vi "List Roots.vi"(8 "Error In":errorcluster, 11 "Tree Manager":T1) -> (0 "Error Out":errorcluster, 1 "Roots IDs":string[](array[string]), 2 "Roots Names":string[](array[string]), 3 "Tree Manager":T1)   [LabVIEW 2016, in "Tree Manager.lvclass"]
doc: "List the Trees that have no Parent ID specified.\n\nThe list order is random."
uses:
  Tree Manager.lvclass
  Typedefs/Session Handle.ctl
  Tree Manager.lvclass/Tree Manager.ctl
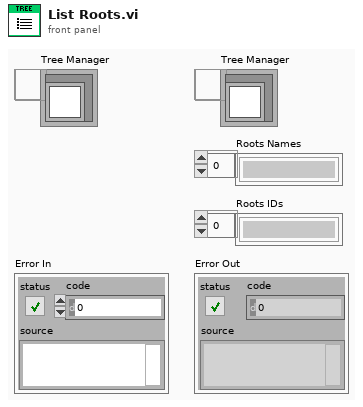
[diagram p1: front panel]
types:
  T1 = typedef "Tree Manager.lvclass/Session Handle.ctl" = refnum<data-value>
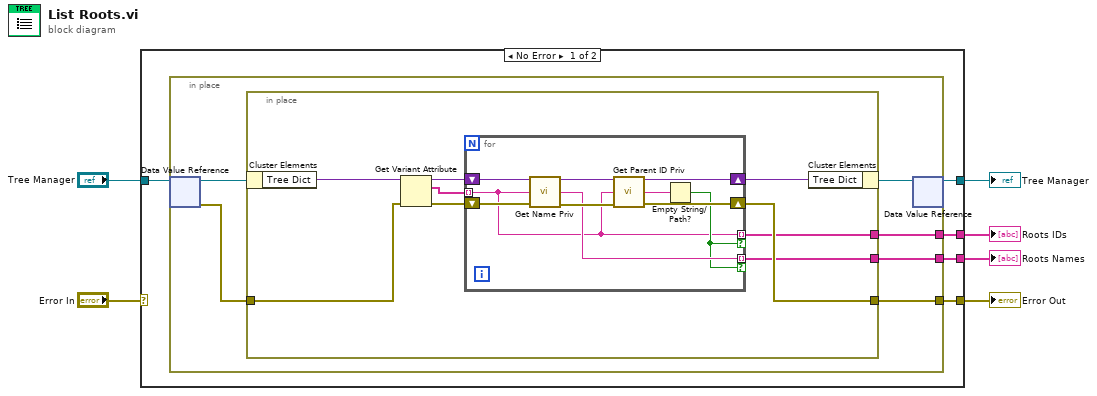
[diagram p0: block diagram]
diagram:
  n1 = case shown="No Error" "Error In" {
    selector: "Error In" -> [_ w37]
    tunnel: "Tree Manager" -> [w11 w38]
    tunnel: [w10 w38] -> w5
    tunnel: [w9 w37] -> w3
    tunnel: [w8 _] -> w2
    tunnel: [w7 _] -> w1
    frame No Error {
      n2 = in-place {
        in-place-border: [w16] -> w9
        in-place-border: [w13] -> w8
        in-place-border: [w12] -> w7
        n3 = in-place-dvr #1(w11) -> (w17:refnum<class "Tree Manager.lvclass">, w14:errorcluster)
        n4 = in-place {
          in-place-border: [w21] -> w16
          in-place-border: w14 -> [w25]
          in-place-border: [w19] -> w13
          in-place-border: [w18] -> w12
          n5 = in-place-cluster #2(w17) -> ("Tree Dict"=w26:variant)
          n6 = Get Variant Attribute(Variant=w26, error in=w25) -> (duplicate Variant=w24:variant, names=w20:string[], error out=w22:errorcluster)  [unwired: 2 in, 1 out]
          n7 = for {
            shift-right: [w36] -> w23
            shift-left: w24 -> [w33]
            shift-right: [w35] -> w21
            shift-left: w22 -> [w30]
            tunnel: w20 -> [w27] mode=indexing
            tunnel: [w27] -> w19 mode=indexing if=w28
            tunnel: [w29] -> w18 mode=indexing if=w28
            n8 = call "Get Name Priv.vi"("Tree Dictionary"=w33, "Unique ID"=w27, "error in"=w30) -> ("Tree Dictionary Out"=w32:variant, "Name"=w29:string, "error out"=w31:errorcluster)  [unwired: 10 in]
            n9 = call "Get Parent ID Priv.vi"("Tree Dictionary"=w32, "Unique ID"=w27, "error in"=w31) -> ("Tree Dictionary Out"=w36:variant, "Parent ID"=w34:string, "error out"=w35:errorcluster)  [unwired: 10 in]
            n10 = Empty String/Path?(string/path=w34) -> (empty?=w28:bool)
          }
          n11 = in-place-cluster #2("Tree Dict"=w23) -> (w15:refnum<class "Tree Manager.lvclass">)
        }
        n12 = in-place-dvr #1(w15) -> (w10:T1)  [unwired: 1 out]
      }
    }
    frame Error {
    }
  }
  "Tree Manager" <- w5
  "Error Out" <- w3
  "Roots IDs" <- w2
  "Roots Names" <- w1
